vi "Fields jsObject Array.vi"(8 "error in (no error)":errorcluster, 9 "FIELDS (none)":T1[](array[typedef]), 10 "Fields jsObject Array Name (\"FIELDS\")":string="FIELDS", 11 "Previous String (\"\")":string) -> (0 "error out":errorcluster, 2 "Fields jsObject Array":string, 3 "Field jsObject Definition":string)   [LabVIEW 2011]
uses:
  Field Record.ctl
  Field DataTypes.ctl
  Field NextItem.ctl
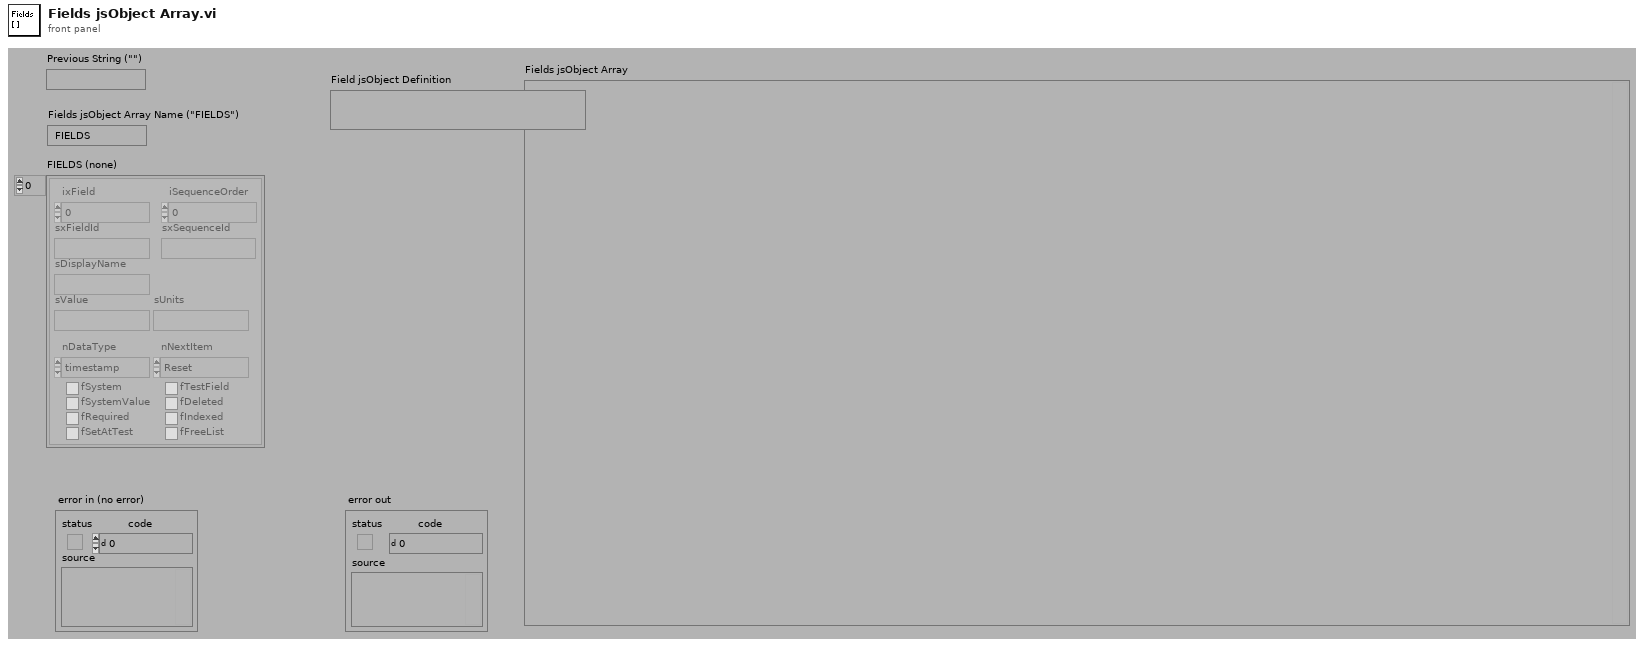
[diagram p1: front panel]
types:
  T1 = typedef "Field Record.ctl" = cluster{"ixField":i32, "iSequenceOrder":i32, "sxFieldId":string, "sxSequenceId":string, "sDisplayName":string, "sValue":string, "sUnits":string, "nDataType":T2, "nNextItem":T3, "fSystem":bool, "fSystemValue":bool, "fRequired":bool, "fSetAtTest":bool, "fTestField":bool, "fDeleted":bool, "fIndexed":bool, "fFreeList":bool}
  T2 = typedef "Field DataTypes.ctl" = enum32{"text", "numeric", "list", "timestamp", "boolean"}
  T3 = typedef "Field NextItem.ctl" = enum32{"Reset", "Retain", "Auto-Increment"}
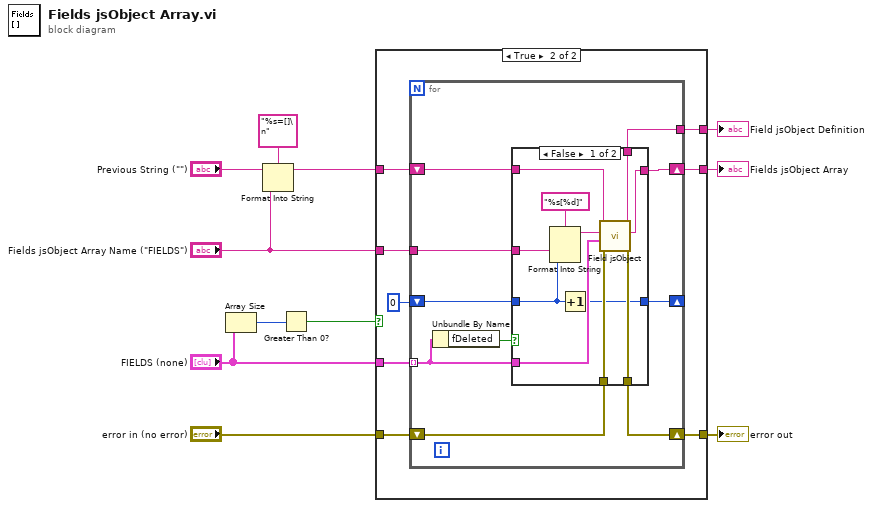
[diagram p0: block diagram]
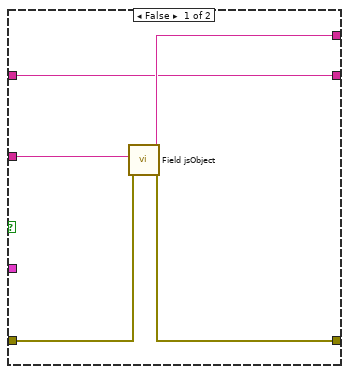
[diagram p2: hidden frame]
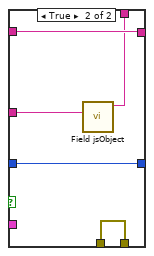
[diagram p3: hidden frame]
diagram:
  n1 = Array Size(array="FIELDS (none)") -> (size(s)=w2:i32)
  n2 = Format Into String(format string="%s=[]\n", initial string="Previous String (\"\")", "Fields jsObject Array Name (\"FIELDS\")") -> (resulting string=w10:string)  [unwired: 1 in, 1 out]
  n3 = Greater Than 0?(x=w2) -> (x > 0?=w1:bool)
  n4 = case shown="True" w1 {
    tunnel: "FIELDS (none)" -> [_ w24]
    tunnel: w10 -> [w12 w23]
    tunnel: "error in (no error)" -> [w16 w22]
    tunnel: [w12 w21] -> w7
    tunnel: [w15 w20] -> w6
    tunnel: "Fields jsObject Array Name (\"FIELDS\")" -> [w13 w19]
    tunnel: [w14 w18] -> w4
    frame False {
      n5 = call "Field jsObject.vi"("error in (no error)"=w16, "Field jsObject Name (\"\")"=w13) -> ("error out"=w15:errorcluster, "Field jsObject Definition"=w14:string)  [unwired: 2 in, 6 out]
    }
    frame True {
      n6 = for {
        tunnel: w24 -> [w27] mode=indexing
        shift-right: [w29] -> w21
        shift-left: w23 -> [w34]
        shift-right: [w32] -> w20
        shift-left: w22 -> [w33]
        tunnel: w19 -> [w31]
        tunnel: [w30] -> w18
        shift-right: [w25] -> _
        shift-left: 0 -> [w28]
        n7 = Unbundle By Name(w27) -> ("fDeleted"=w26:bool)
        n8 = case shown="False" w26 {
          tunnel: w34 -> [w45 w48]
          tunnel: w27 -> [w44 _]
          tunnel: w33 -> [w43 w49]
          tunnel: [w42 w49] -> w32
          tunnel: w31 -> [w39 w47]
          tunnel: [w38 w46] -> w30
          tunnel: [w37 w48] -> w29
          tunnel: w28 -> [w36 w50]
          tunnel: [w35 w50] -> w25
          frame False {
            n9 = Format Into String(format string="%s[%d]", w39, w36) -> (resulting string=w40:string)  [unwired: 2 in, 1 out]
            n10 = Increment(x=w36) -> (x+1=w35:i32)
            n11 = call "Field jsObject.vi"("error in (no error)"=w43, "Field Record (empty)"=w44, "Field jsObject Name (\"\")"=w40, "Previous String (\"\")"=w45) -> ("error out"=w42:errorcluster, "Field jsObject"=w37:string, "Field jsObject Definition"=w38:string)  [unwired: 5 out]
          }
          frame True {
            n12 = call "Field jsObject.vi"("Field jsObject Name (\"\")"=w47) -> ("Field jsObject Definition"=w46:string)  [unwired: 3 in, 7 out]
          }
        }
      }
    }
  }
  "Fields jsObject Array" <- w7
  "error out" <- w6
  "Field jsObject Definition" <- w4
